vi "getSpecificElement.vi"(8 "error in (no error)":errorcluster, 10 "nameElem":string, 11 "Topic in":refnum<class "Topic.lvclass">) -> (0 "error out":errorcluster, 2 "Element.lvclass":refnum<class "Element.lvclass">, 3 "Topic out":refnum<class "Topic.lvclass">)   [LabVIEW 2018, in "Topic.lvclass"]
doc: "Get the specific element based on the element's name."
uses:
  Topic.lvclass
  Element/Element.lvclass
  Topic.lvclass/Topic.ctl
  Element/Element.lvclass/Element.ctl
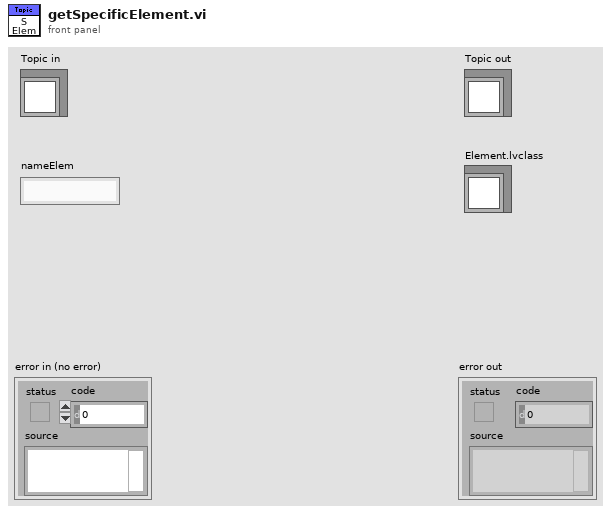
[diagram p1: front panel]
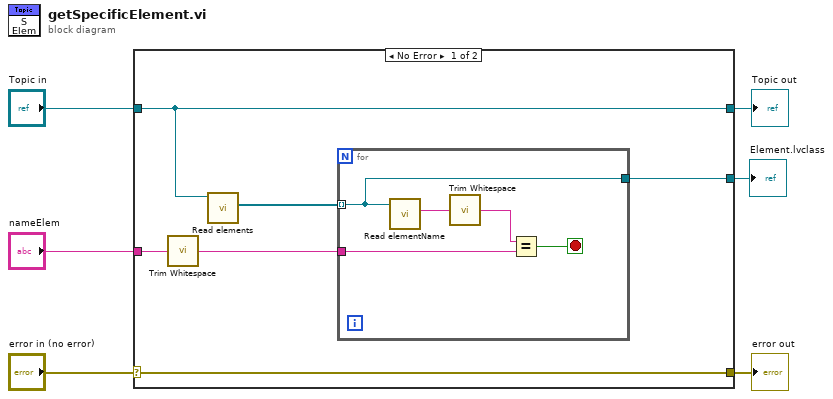
[diagram p0: block diagram]
diagram:
  n1 = case shown="No Error" "error in (no error)" {
    selector: "error in (no error)" -> [w12 w19]
    tunnel: [w12 w19] -> w5
    tunnel: [w10 w18] -> w3
    tunnel: "Topic in" -> [w10 w18]
    tunnel: "nameElem" -> [w11 _]
    tunnel: [w7 _] -> w1
    frame No Error {
      n2 = call <vilib>:"Trim Whitespace.vi"("string"=w11) -> ("trimmed string"=w9:string)  [unwired: 1 in]
      n3 = call "Read elements.vi"("Topic in"=w10) -> ("elements"=w8:refnum<class "Element.lvclass">[])  [unwired: 8 in, 2 out]
      n4 = for {
        tunnel: w9 -> [w15]
        tunnel: w8 -> [w13] mode=indexing
        tunnel: [w13] -> w7
        stop <- w17 stop-if-true
        n5 = call "Read elementName.vi"("Element in"=w13) -> ("elementName"=w14:string)  [unwired: 8 in, 2 out]
        n6 = call <vilib>:"Trim Whitespace.vi"("string"=w14) -> ("trimmed string"=w16:string)  [unwired: 1 in]
        n7 = Equal?(x=w16, y=w15) -> (x = y?=w17:bool)
      }
    }
    frame Error {
    }
  }
  "error out" <- w5
  "Topic out" <- w3
  "Element.lvclass" <- w1
